vi "Write Waveform.vi"(8 "error in (no error)":errorcluster, 10 "I-V parameters":T1={"Start magnitude"=0.001, "Magnitude increment"=0.001, "End magnitude"=0.01, "Ramp length"=0, "Top  length"=0, "Threshold "=2e-06, "Processing delay"=0, "Valhalla range"=0.001, "Interpolation"=64, "Stop after"=1, "Detector window"=480} {"Detector window" format="%dpts"; "Stop after" format="%d sweep(s)"; "Valhalla range" format="%#_6pA"; "Processing delay" format="%dpts"; "Threshold" format="%#_6pV"; "Top  length" format="%dpts"; "Ramp length" format="%dpts"; "End magnitude" format="%#_6pA"; "Magnitude increment" format="%#_6pA"; "Start magnitude" format="%#_6pA"}, 11 "RP Communicator in":refnum<class "RP Communicator.lvclass">) -> (0 "error out":errorcluster, 2 "Output Waveform":i16[](graph), 3 "RP Communicator out":refnum<class "RP Communicator.lvclass">)   [LabVIEW 2016, in "RP Communicator.lvclass"]
uses:
  RP Communicator.lvclass
  Waform generation/I-V parameters.ctl
  RP Communicator.lvclass/RP Communicator.ctl
panel:
  # "Waveform parameters"
  # "Detector parameters"
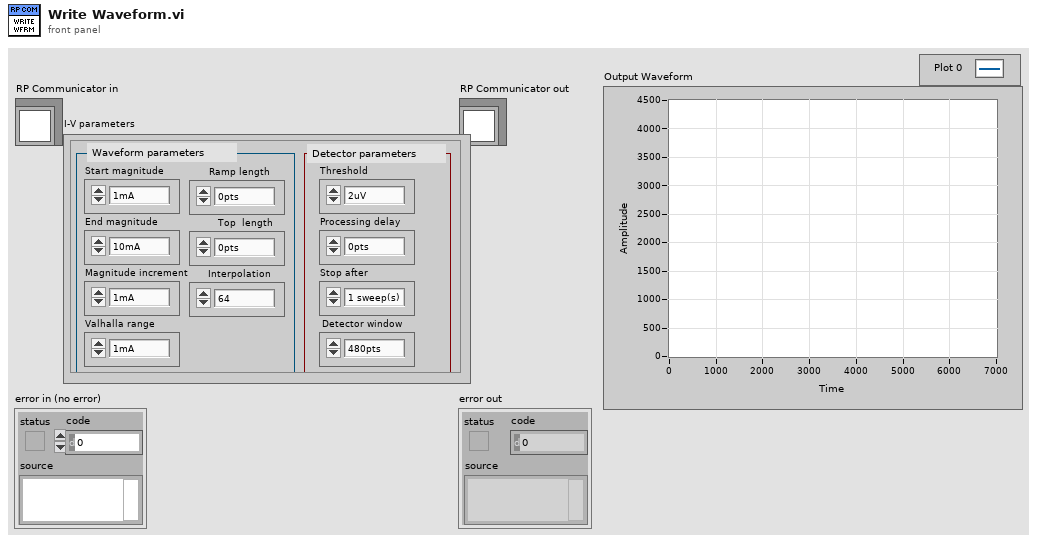
[diagram p1: front panel]
types:
  T1 = typedef "I-V parameters.ctl" = cluster{"Start magnitude":dbl, "Magnitude increment":dbl, "End magnitude":dbl, "Ramp length":i32, "Top  length":i32, "Threshold ":dbl, "Processing delay":u16, "Valhalla range":dbl, "Interpolation":i32, "Stop after":u16, "Detector window":i32}
  T2 = typedef "Waveform parameters.ctl" = cluster{"Start magnitude":dbl, "Magnitude increment":dbl, "Number of pulses":i32, "Ramp length":i32, "Top  length":i32, "Threshold ":i32, "Processing delay":u16, "Stop after":u16, "Detector window":i32}
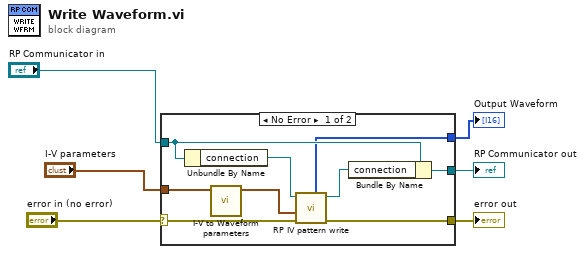
[diagram p0: block diagram]
diagram:
  n1 = case shown="No Error" "error in (no error)" {
    selector: "error in (no error)" -> [w11 w17]
    tunnel: [w10 w17] -> w5
    tunnel: [w9 w16] -> w3
    tunnel: "RP Communicator in" -> [w14 w16]
    tunnel: "I-V parameters" -> [w15 _]
    tunnel: [w7 _] -> w1
    frame No Error {
      n2 = Unbundle By Name(w14) -> ("connection"=w13:refnum<k5>)
      n3 = call "I-V to Waveform parameters.vi"("I-V parameters"=w15) -> ("Waveform parameters out"=w12:T2)  [unwired: 10 in]
      n4 = call "RP IV pattern write.vi"("Error In"=w11, "Waveform parameters"=w12, "connection ID"=w13) -> ("Error Out"=w10:errorcluster, "connection ID out"=w8:refnum<k5>, "Waveform Graph"=w7:i16[])  [unwired: 6 in]
      n5 = Bundle By Name(cluster=w14, "connection"=w8) -> (w9:refnum<class "RP Communicator.lvclass">)
    }
    frame Error {
    }
  }
  "error out" <- w5
  "RP Communicator out" <- w3
  "Output Waveform" <- w1
